vi "sequencetest.vi"() -> ()   [LabVIEW 2009]
panel:
  in  "OK Button":bool
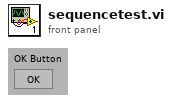
[diagram p1: front panel]
types:
  T1 = typedef "IMAQ Image.ctl" = refnum<image>
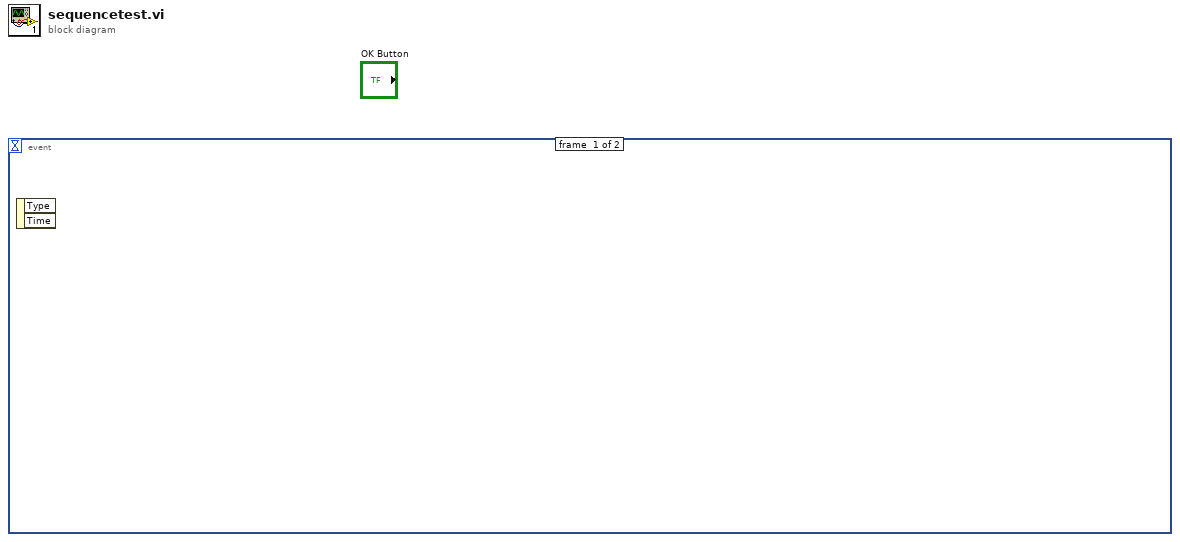
[diagram p0: block diagram]
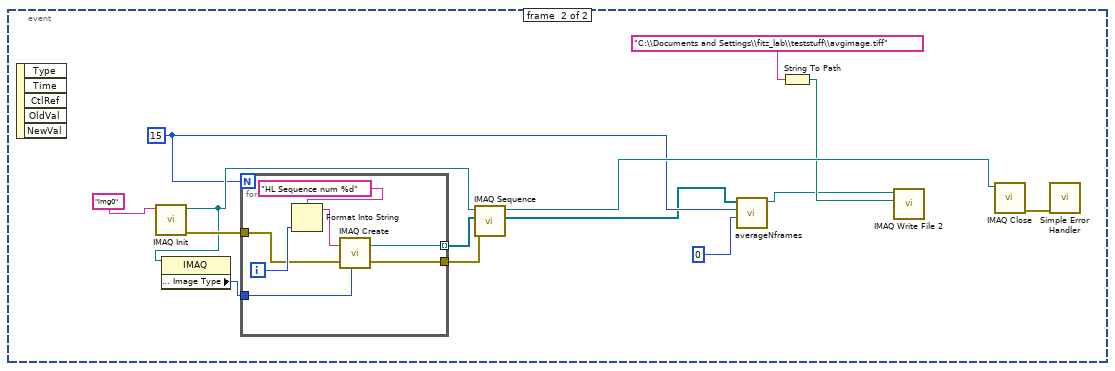
[diagram p2: hidden frame]
diagram:
  n1 = event shown="[1] \"OK Button\": Value Change" {
    selector: _ -> [_ _]
    dyn-events: _ -> [_ _]
    timeout: _ -> [_ _]
    event #0 {
      n2 = event-data() -> ()  [unwired: 1 in, 2 out]
    }
    event #1 {
      w4 = 15
      n3 = event-data() -> ()  [unwired: 1 in, 5 out]
      n4 = call <vilib>:"IMAQ Init.vi"("Interface Name"="img0") -> ("error out"=w11:errorcluster, "IMAQ Session Out"=w10:refnum<k11>)  [unwired: 9 in]
      n5 = property class="IMAQ"(reference=w10) -> ("Image Parameters : Image Type"=w8:u32)  [unwired: 1 in, 2 out]
      n6 = for {
        N: w4 -> [_]
        tunnel: w8 -> [w18]
        tunnel: [w17] -> w9 mode=indexing
        tunnel: w11 -> [w16]
        tunnel: [w15] -> w12
        i -> [w21]
        n7 = Format Into String(format string="HL Sequence num %d", w21) -> (resulting string=w19:string)  [unwired: 2 in, 1 out]
        n8 = call "IMAQ Create"("Image Name"=w19, "Image Type"=w18, "error in (no error)"=w16) -> ("New Image"=w17:T1, "error out"=w15:errorcluster)  [unwired: 2 in]
      }
      n9 = call <vilib>:"IMAQ Sequence.vi"("error in (no error)"=w12, "Images In"=w9, "IMAQ Session In"=w10) -> ("Images Out"=w3:T1[], "IMAQ Session Out"=w6:refnum<k11>)  [unwired: 6 in, 1 out]
      n10 = call "averageNframes.vi"("first frame index"=0, "number of frames"=w4, "Images In"=w3) -> ("Image out"=w1:T1)  [unwired: 8 in]
      n11 = String To Path(string="C:\\Documents and Settings\\fitz_lab\\teststuff\\avgimage.tiff") -> (path=w2:path)
      n12 = call-poly "IMAQ Write File 2"("File Path"=w2, "Image"=w1) -> ()  [unwired: 8 in, 2 out]
      n13 = call <vilib>:"IMAQ Close.vi"("IMAQ Session In"=w6) -> ("error out"=w14:errorcluster)  [unwired: 10 in]
      n14 = call <vilib>:"Simple Error Handler.vi"("error in (no error)"=w14) -> ()  [unwired: 4 in, 5 out]
    }
  }
